vi "2-D_CircularBuffer.vi"(6 "DataIn":dbl[](array[numeric]), 8 "ErrorIn":errorcluster, 9 "BufferSize#Columns":i32=10000, 10 "BufferSize#Rows":i32=4, 11 "Mode":T1) -> (0 "ErrorOut":errorcluster, 3 "DataOut":dbl[][](array[numeric]), 4 "BufferOut":dbl[][](array[numeric]))   [LabVIEW 2018]
doc: "This VI allows for the creation, update and Reading of a 2-D Circular Buffer\n\nCopyright © 2011 Epimedia, Inc. All Rights Reserved.\n\nThe Epimedia Application Library is Copyright © 2009-2011 Epimedia, Inc. \nAll Rights Reserved. Used under license.s"
uses:
  Controls/2-D_CircularBufferModeEnum.ctl
panel:
  # "Copyright © 2011 Epimedia, Inc. All Rights Reserved.\n\nThe Epimedia Application Library is Copyright © 2009-2011 Epimedia, Inc. \nAll Rights Reserved. Used under license."
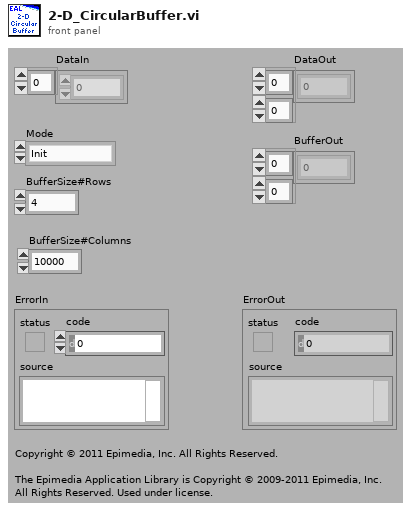
[diagram p1: front panel]
types:
  T1 = typedef "2-D_CircularBufferModeEnum.ctl" = enum16{"Init", "AddData", "Read"}
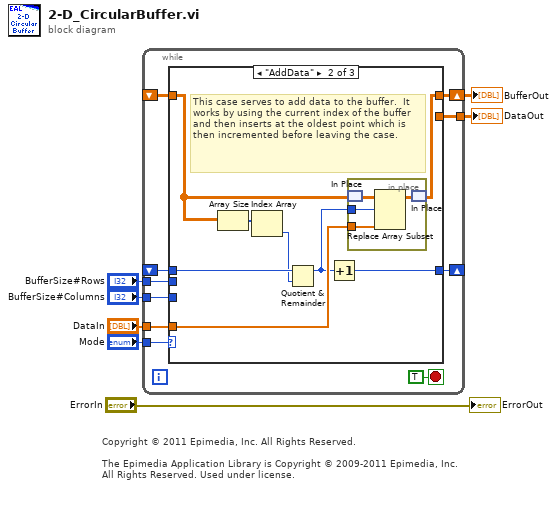
[diagram p0: block diagram]
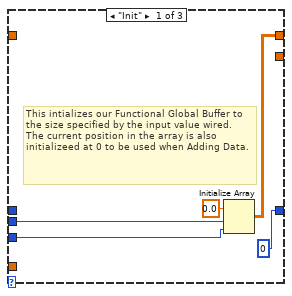
[diagram p2: hidden frame]
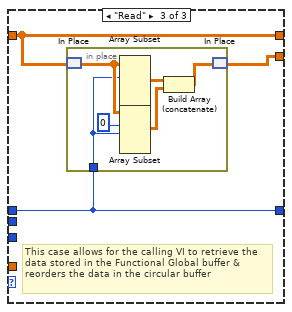
[diagram p3: hidden frame]
diagram:
  # "Copyright © 2011 Epimedia, Inc. All Rights Reserved.\n\nThe Epimedia Application Library is Copyright © 2009-2011 Epimedia, Inc. \nAll Rights Reserved. Used under license."
  n1 = while {
    tunnel: "Mode" -> [w16]
    shift-right: [w15] -> w1
    shift-left: _ -> [w13]
    tunnel: "DataIn" -> [w14]
    tunnel: "BufferSize#Rows" -> [w12]
    shift-right: [w11] -> _
    shift-left: _ -> [w10]
    tunnel: "BufferSize#Columns" -> [w9]
    tunnel: [w8] -> w2
    stop <- TRUE stop-if-true
    n2 = case shown="\"AddData\"" w16 {
      tunnel: [w21 w30 w36] -> w15
      tunnel: w14 -> [_ w29 _]
      tunnel: w13 -> [_ w26 w36]
      tunnel: w12 -> [w20 _ _]
      tunnel: [0 ("BufferSize#Columns") w27 w37] -> w11
      tunnel: w10 -> [_ w28 w37]
      tunnel: w9 -> [w18 _ _]
      tunnel: [_ _ w35] -> w8
      frame "Init" {
        # "This intializes our Functional Global Buffer to the size specified by the input value wired.  The current position in the array is also initializeed at 0 to be used when Adding Data."
        n3 = Initialize Array(0.0 ("Numeric"), w20, w18) -> (w21:dbl[][])
      }
      frame "AddData" {
        # "This case serves to add data to the buffer.  It works by using the current index of the buffer and then inserts at the oldest point which is then incremented before leaving the case."
        n4 = Array Size(array=w26) -> (size(s)=w25:i32[])
        n5 = Index Array(array=w25) -> (element=w24:i32)  [unwired: 1 in]
        n6 = Quotient & Remainder(x=w28, y=w24) -> (x-y*floor(x/y)=w23:i32)  [unwired: 1 out]
        n7 = Increment(x=w23) -> (x+1=w27:i32)
        n8 = in-place {
          in-place-border: w29 -> [w34]
          in-place-border: w23 -> [w32]
          n9 = in-place-match #1(w26) -> (w31:dbl[][])
          n10 = Replace Array Subset(array=w31, new element=w34, index (row)=w32) -> (w33:dbl[][])  [unwired: 1 in]
          n11 = in-place-match #1(w33) -> (w30:dbl[][])
        }
      }
      frame "Read" {
        # "This case allows for the calling VI to retrieve the data stored in the Functional Global buffer & reorders the data in the circular buffer"
        n12 = in-place {
          in-place-border: w37 -> [w38]
          n13 = in-place-match #2(w36) -> (w42:dbl[][])
          n14 = Array Subset(array=w42, index (row)=w38) -> (w40:dbl[][])  [unwired: 3 in]
          n15 = Array Subset(array=w42, index (row)=0 ("index"), length (row)=w38) -> (w39:dbl[][])  [unwired: 2 in]
          n16 = Build Array (concatenate)(w40, w39) -> (w41:dbl[][])
          n17 = in-place-match #2(w41) -> (w35:dbl[][])
        }
      }
    }
  }
  "DataOut" <- w2
  "BufferOut" <- w1
  "ErrorOut" <- "ErrorIn"
